vi "Read Device Information.vi"(8 "error in (no error)":errorcluster, 11 "TroSpec in":refnum<class "PL ISTEQ TroSpec.lvclass">) -> (0 "error out":errorcluster, 2 "device information":T1 {"max period, s" format="%#_6p"; "min period, s" format="%#_6p"; "CCD type" items=["Toshiba TCD1304AP"=1, "Hamamatsu G11620-512DA"=2, "Hamamatsu 3901-512Q"=3]}, 3 "TroSpec out":refnum<class "PL ISTEQ TroSpec.lvclass">)   [LabVIEW 2015, in "PL ISTEQ TroSpec.lvclass"]
doc: "Reads device information."
uses:
  PL ISTEQ TroSpec.lvclass
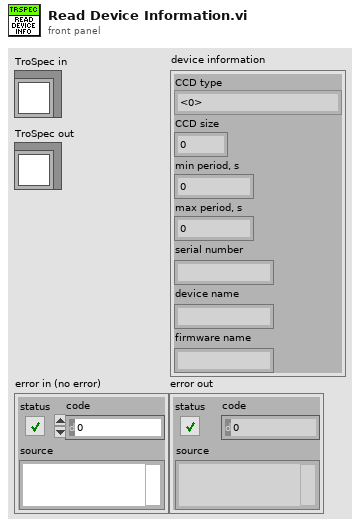
[diagram p1: front panel]
types:
  T1 = cluster{"CCD type":u16, "CCD size":u16, "min period, s":dbl, "max period, s":dbl, "serial number":string, "device name":string, "firmware name":string}
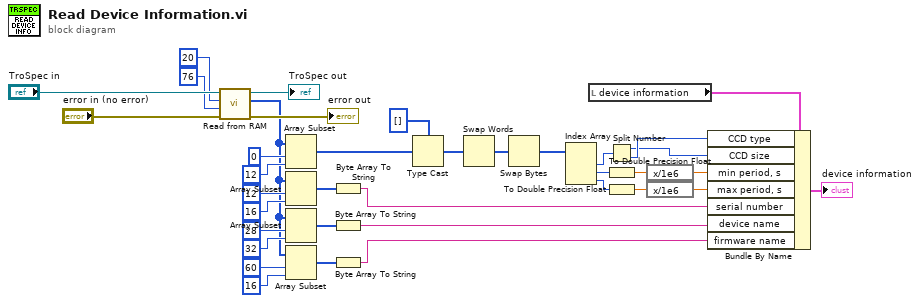
[diagram p0: block diagram]
diagram:
  n1 = call "Read from RAM.vi"("error in (no error)"="error in (no error)", "size"=u16 76, "address"=u16 20, "TroSpec in"="TroSpec in") -> ("error out"=→"error out":errorcluster, "data"=w22:u8[], "TroSpec out"=→"TroSpec out":refnum<class "PL ISTEQ TroSpec.lvclass">)  [unwired: 5 in]
  n2 = Array Subset(array=w22, index=0, length=12) -> (w21:u8[])
  n3 = Array Subset(array=w22, index=12, length=16) -> (w14:u8[])
  n4 = Array Subset(array=w22, index=28, length=32) -> (w13:u8[])
  n5 = Array Subset(array=w22, index=60, length=16) -> (w12:u8[])
  n6 = Byte Array To String(unsigned byte array=w14) -> (string=w9:string)
  n7 = Byte Array To String(unsigned byte array=w13) -> (string=w10:string)
  n8 = Byte Array To String(unsigned byte array=w12) -> (string=w11:string)
  n9 = Type Cast(type=u32[] [] ("data"), x=w21) -> (*(type *) &x=w19:u32[])
  n10 = Swap Words(1:w19) -> (0:w20:u32[])
  n11 = Swap Bytes(anything=w20) -> (byte swapped=w17:u32[])
  n12 = Index Array(array=w17) -> (element #1=w8:u32, element #2=w16:u32, element #3=w15:u32)  [unwired: 3 in]
  n13 = local read "device information"() -> (w31:T1)
  n14 = Split Number(x=w8) -> (hi(x)=w6:u16, lo(x)=w7:u16)
  n15 = To Double Precision Float(number=w16) -> (double precision float=w4:dbl)
  n16 = To Double Precision Float(number=w15) -> (double precision float=w2:dbl)
  n17 = expression code="x/1e6"(w4) -> (w3:dbl)
  n18 = expression code="x/1e6"(w2) -> (w1:dbl)
  n19 = Bundle By Name(cluster=w31, "CCD type"=w7, "CCD size"=w6, "min period, s"=w3, "max period, s"=w1, "serial number"=w9, "device name"=w10, "firmware name"=w11) -> (→"device information":T1)
